vi "AVS_GetDigIn.vi"(0 "a_hDevice":i32, 7 "a_DigInId":u8, 11 "a_pDigIn":u8) -> (4 "Output Value":i32, 15 "a_pDigIn":u8)   [LabVIEW 2018]
uses:
  avaspecx64.dll
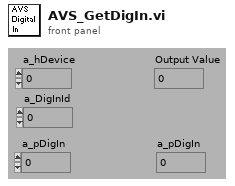
[diagram p1: front panel]
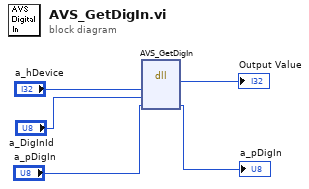
[diagram p0: block diagram]
diagram:
  n1 = dll-call lib="C:/AvaSpecX64-DLL_9.7/examples/LabView/LabViewSingleChan/avaspecx64.dll" fn="AVS_GetDigIn"("a_hDevice"="a_hDevice", "a_DigInId"="a_DigInId", "a_pDigIn"="a_pDigIn") -> ("return type"=→"Output Value":i32, "a_pDigIn"=→"a_pDigIn":u8)  [unwired: 5 in, 2 out]
